vi "Global 1.vi"() -> ()   [LabVIEW 2024]
panel:
  in  "Temperature (ADC)":u8
  in  "Fan speed (ADC)":u8
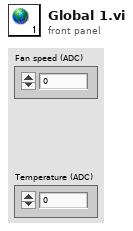
[diagram p1: front panel]
diagram:
